vi "get write location.vi"() -> ()   [LabVIEW 2010]
panel:
  out "3D write location":u32
  out "2D index":u32
  in  "reader status":T1
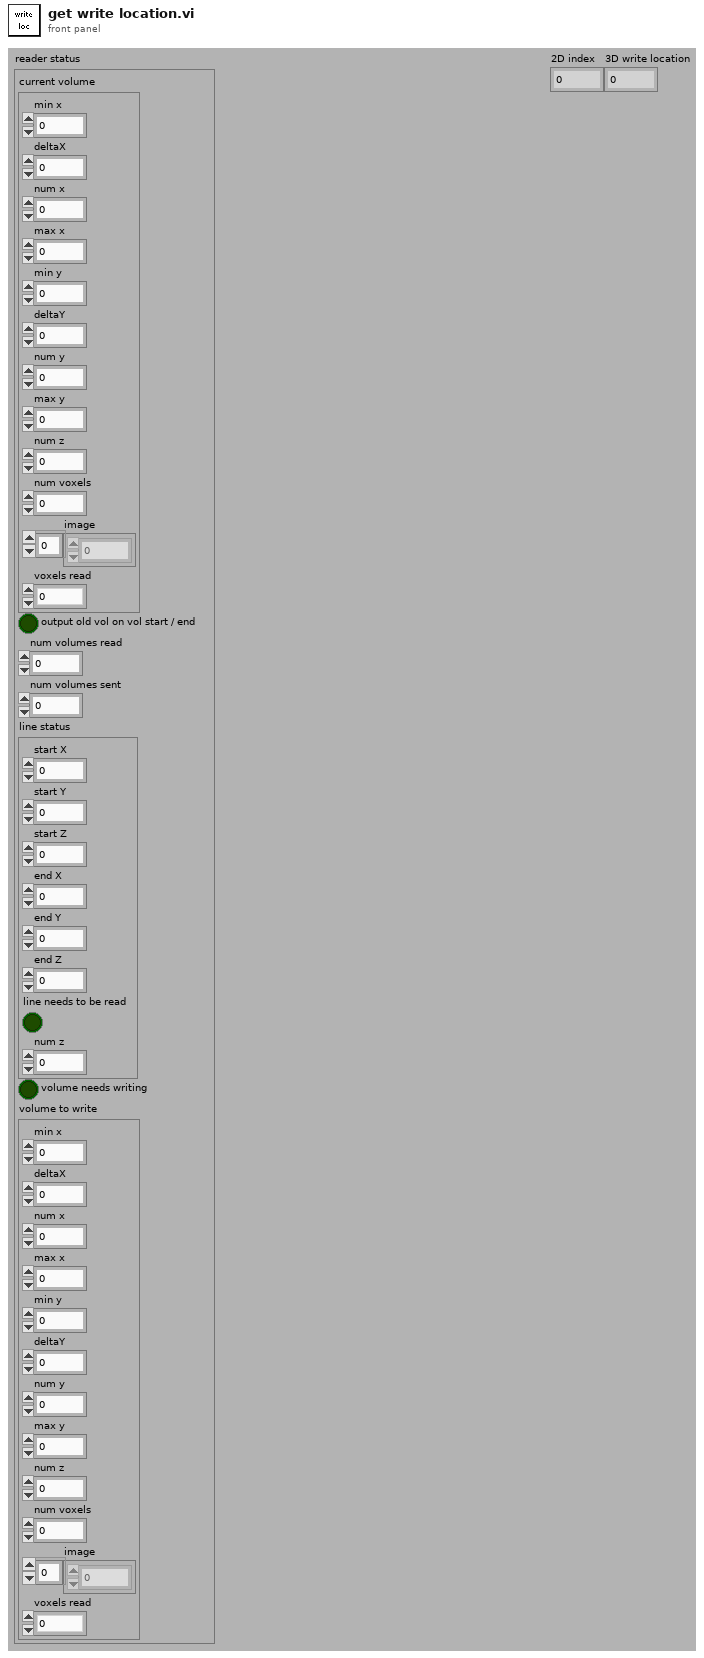
[diagram p1: front panel]
types:
  T1 = cluster{"current volume":cluster{"min x":i16, "deltaX":dbl, "num x":u32, "max x":i16, "min y":i16, "deltaY":dbl, "num y":u32, "max y":i16, "num z":u32, "num voxels":u32, "image":u32[], "voxels read":u32}, "output old vol on vol start / end":bool, "num volumes read":u32, "num volumes sent":u32, "line status":cluster{"start X":i16, "start Y":i16, "start Z":i16, "end X":i16, "end Y":i16, "end Z":i16, "line needs to be read":bool, "num z":u8}, "volume needs writing":bool, "volume to write":cluster{"min x":i16, "deltaX":dbl, "num x":u32, "max x":i16, "min y":i16, "deltaY":dbl, "num y":u32, "max y":i16, "num z":u32, "num voxels":u32, "image":u32[], "voxels read":u32}}
  T2 = cluster{"start X":i16, "start Y":i16, "start Z":i16, "end X":i16, "end Y":i16, "end Z":i16, "line needs to be read":bool, "num z":u8}
  T3 = cluster{"min x":i16, "deltaX":dbl, "num x":u32, "max x":i16, "min y":i16, "deltaY":dbl, "num y":u32, "max y":i16, "num z":u32, "num voxels":u32, "image":u32[], "voxels read":u32}
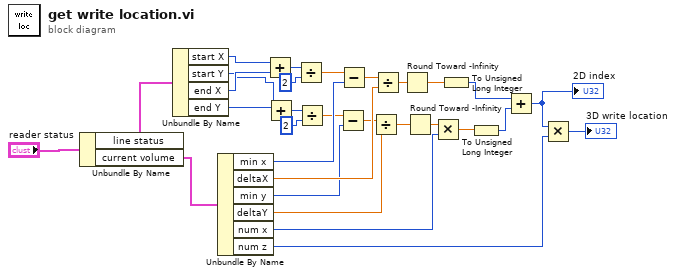
[diagram p0: block diagram]
diagram:
  n1 = Unbundle By Name("reader status") -> ("line status"=w28:T2, "current volume"=w29:T3)
  n2 = Unbundle By Name(w28) -> ("start X"=w27:i16, "start Y"=w21:i16, "end X"=w26:i16, "end Y"=w20:i16)
  n3 = Unbundle By Name(w29) -> ("min x"=w18:i16, "deltaX"=w16:dbl, "min y"=w13:i16, "deltaY"=w11:dbl, "num x"=w8:u32, "num z"=w2:u32)
  n4 = Add(x=w27, y=w26) -> (x+y=w25:i16)
  n5 = Add(x=w21, y=w20) -> (x+y=w23:i16)
  n6 = Divide(x=w25, y=i16 2) -> (x/y=w19:dbl)
  n7 = Divide(x=w23, y=i16 2) -> (x/y=w14:dbl)
  n8 = Subtract(x=w14, y=w13) -> (x-y=w12:dbl)
  n9 = Subtract(x=w19, y=w18) -> (x-y=w17:dbl)
  n10 = Divide(x=w12, y=w11) -> (x/y=w10:dbl)
  n11 = Divide(x=w17, y=w16) -> (x/y=w15:dbl)
  n12 = Round Toward -Infinity(1:w15) -> (0:w7:dbl)
  n13 = Round Toward -Infinity(1:w10) -> (0:w9:dbl)
  n14 = Multiply(x=w9, y=w8) -> (x*y=w6:dbl)
  n15 = To Unsigned Long Integer(number=w7) -> (unsigned 32bit integer=w5:u32)
  n16 = To Unsigned Long Integer(number=w6) -> (unsigned 32bit integer=w4:u32)
  n17 = Add(x=w5, y=w4) -> (x+y=w3:u32)
  "2D index" <- w3
  n18 = Multiply(x=w3, y=w2) -> (x*y=→"3D write location":u32)
